vi "ReadEXCEL.vi"(8 "错误输入（无错误）":errorcluster, 9 "EXCEL 标签":string="Sheet1", 10 "路径":path) -> (0 "错误输出":errorcluster, 1 "数据":string[][](array[string]))   [LabVIEW 2018]
panel:
  in  "数组":string[][](array[string])
  in  "Excel._Worksheet":refnum<k7>
  in  "Excel._Application":refnum<k7>
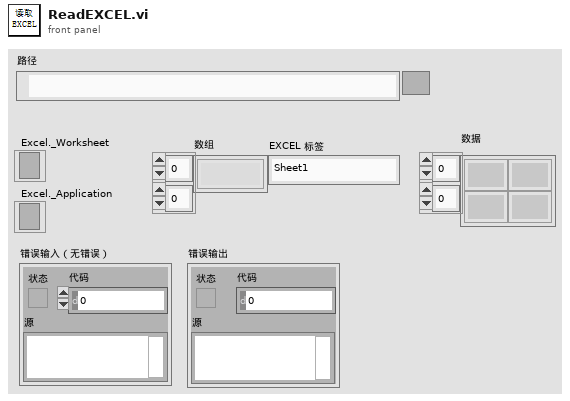
[diagram p1: front panel]
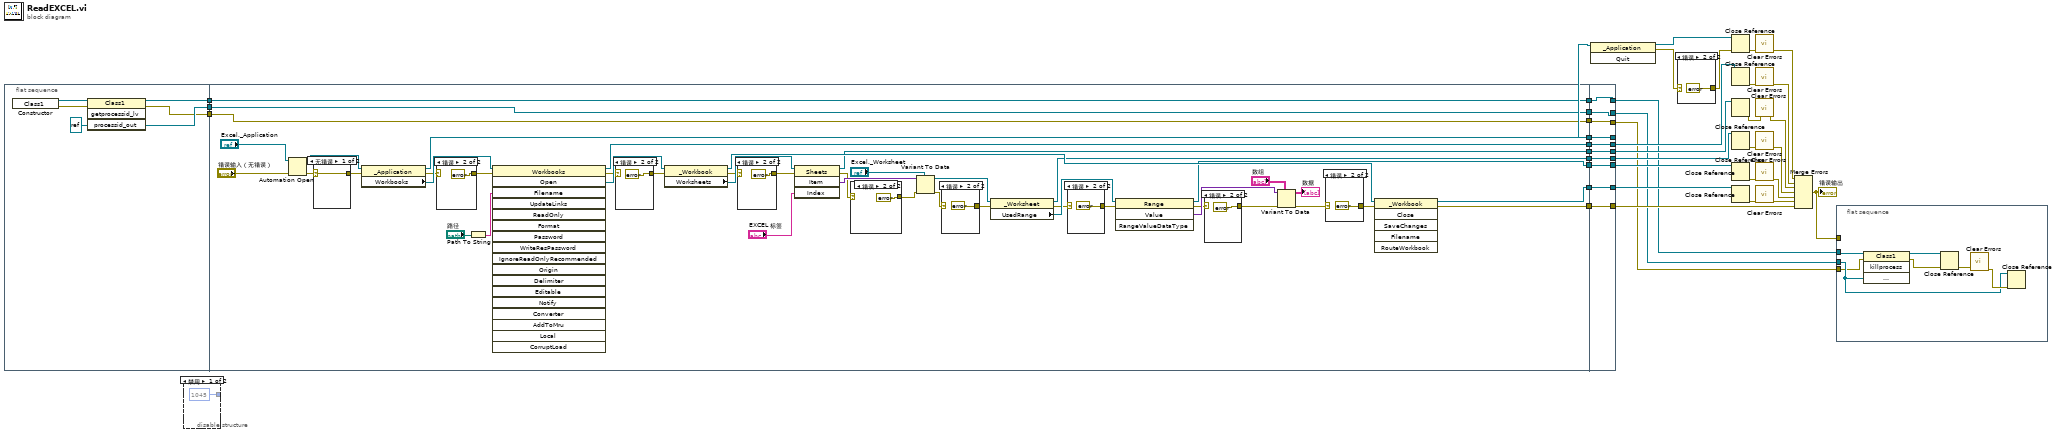
[diagram p0: block diagram]
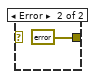
[diagram p11: hidden frame]
diagram:
  n1 = flat-sequence {
    tunnel: [w43] -> w11
    tunnel: [w42] -> w10
    tunnel: [w40] -> w3
    tunnel: [w75] -> w18
    tunnel: [w74] -> w17
    tunnel: [w73] -> w16
    tunnel: [w68] -> w15
    tunnel: [w70] -> w14
    tunnel: [w72] -> w13
    tunnel: [w71] -> w12
    tunnel: w11 -> [w47]
    tunnel: w10 -> [w48]
    tunnel: [w48] -> w9
    tunnel: [w47] -> w8
    tunnel: [w46] -> w4
    tunnel: w3 -> [w46]
    tunnel: [w112] -> w22
    tunnel: [w113] -> w29
    tunnel: [w114] -> w1
    tunnel: [w115] -> w31
    tunnel: [w116] -> w33
    tunnel: [w117] -> w35
    tunnel: [w118] -> w36
    tunnel: w18 -> [w118]
    tunnel: w17 -> [w117]
    tunnel: w16 -> [w116]
    tunnel: w15 -> [w115]
    tunnel: w14 -> [w114]
    tunnel: w13 -> [w113]
    tunnel: w12 -> [w112]
    tunnel: [w111] -> w5
    tunnel: w9 -> [w111]
    tunnel: [w110] -> w6
    tunnel: w8 -> [w110]
    tunnel: [w109] -> w2
    tunnel: w4 -> [w109]
    frame #0 {
      n2 = constructor class="Class1"() -> (reference out=w45:refnum<k24>, error out=w41:errorcluster)  [unwired: 3 in, 1 out]
      n3 = invoke on="调用节点" class="Class1" method="getprocessid_lv"(reference=w45, error in=w41, "processid_out"=refnum<k24> refnum) -> (reference out=w43:refnum<k24>, error out=w40:errorcluster, "processid_out"=w42:refnum<k24>)  [unwired: 1 in, 1 out]
    }
    frame #1 {
      n4 = Automation Open(error in (no error)="错误输入（无错误）", Automation Refnum="Excel._Application") -> (Automation Refnum=w69:refnum<k7>, error out=w66:errorcluster)  [unwired: 2 out]
      n5 = case shown="无错误" w66 {
        selector: w66 -> [w107 _]
        tunnel: [w107 errorcluster {"status"=FALSE, "code"=0, "source"=""} ("error IO")] -> w65
        frame No Error {
        }
        frame Error {
        }
      }
      n6 = property class="_Application"(reference=w69, error in=w65) -> (reference out=w70:refnum<k7>, error out=w64:errorcluster, "Workbooks"=w67:refnum<k7>)
      n7 = case shown="错误" w64 {
        selector: w64 -> [w105 _]
        tunnel: [w105 errorcluster {"status"=FALSE, "code"=0, "source"=""} ("error IO")] -> w63
        frame No Error {
        }
        frame Error {
        }
      }
      n8 = Path To String(path="路径") -> (string=w79:string)
      n9 = invoke class="Workbooks" method="Open"(reference=w67, error in=w63, "Filename"=w79) -> (reference out=w68:refnum<k7>, error out=w62:errorcluster, "Open"=w90:refnum<k7>)  [unwired: 15 in, 15 out]
      n10 = case shown="错误" w62 {
        selector: w62 -> [w103 _]
        tunnel: [w103 errorcluster {"status"=FALSE, "code"=0, "source"=""} ("error IO")] -> w61
        frame No Error {
        }
        frame Error {
        }
      }
      n11 = property class="_Workbook"(reference=w90, error in=w61) -> (reference out=w78:refnum<k7>, error out=w60:errorcluster, "Worksheets"=w89:refnum<k7>)
      n12 = case shown="错误" w60 {
        selector: w60 -> [w101 _]
        tunnel: [w101 errorcluster {"status"=FALSE, "code"=0, "source"=""} ("error IO")] -> w59
        frame No Error {
        }
        frame Error {
        }
      }
      n13 = invoke class="Sheets" method="Item"(reference=w89, error in=w59, "Index"="EXCEL 标签") -> (reference out=w73:refnum<k7>, error out=w58:errorcluster, "Item"=w88:variant)  [unwired: 1 in, 1 out]
      n14 = case shown="错误" w58 {
        selector: w58 -> [w99 _]
        tunnel: [w99 errorcluster {"status"=FALSE, "code"=0, "source"=""} ("error IO")] -> w57
        frame No Error {
        }
        frame Error {
        }
      }
      n15 = Variant To Data(error in=w57, type="Excel._Worksheet", Variant=w88) -> (data=w86:refnum<k7>, error out=w56:errorcluster)
      n16 = case shown="错误" w56 {
        selector: w56 -> [w97 _]
        tunnel: [w97 errorcluster {"status"=FALSE, "code"=0, "source"=""} ("error IO")] -> w55
        frame No Error {
        }
        frame Error {
        }
      }
      n17 = property class="_Worksheet"(reference=w86, error in=w55) -> (reference out=w74:refnum<k7>, error out=w54:errorcluster, "UsedRange"=w85:refnum<k7>)
      n18 = case shown="错误" w54 {
        selector: w54 -> [w95 _]
        tunnel: [w95 errorcluster {"status"=FALSE, "code"=0, "source"=""} ("error IO")] -> w53
        frame No Error {
        }
        frame Error {
        }
      }
      n19 = invoke class="Range" method="Value"(reference=w85, error in=w53) -> (reference out=w75:refnum<k7>, error out=w52:errorcluster, "Value"=w84:variant)  [unwired: 2 in, 1 out]
      n20 = case shown="错误" w52 {
        selector: w52 -> [w93 _]
        tunnel: [w93 errorcluster {"status"=FALSE, "code"=0, "source"=""} ("error IO")] -> w51
        frame No Error {
        }
        frame Error {
        }
      }
      n21 = Variant To Data(error in=w51, type="数组", Variant=w84) -> (data=→"数据":string[][], error out=w50:errorcluster)
      n22 = case shown="错误" w50 {
        selector: w50 -> [w91 _]
        tunnel: [w91 errorcluster {"status"=FALSE, "code"=0, "source"=""} ("error IO")] -> w49
        frame No Error {
        }
        frame Error {
        }
      }
      n23 = invoke class="_Workbook" method="Close"(reference=w78, error in=w49) -> (reference out=w72:refnum<k7>, error out=w71:errorcluster)  [unwired: 4 in, 4 out]
    }
    frame #2 {
    }
  }
  n24 = disable-structure shown="禁用" {
    disable-tunnel: [1045 ("specific error code to clear (0: all)") _] -> _
    frame Disabled {
    }
    frame Enabled {
    }
  }
  n25 = invoke class="_Application" method="Quit"(reference=w1) -> (reference out=w21:refnum<k7>, error out=w20:errorcluster)  [unwired: 2 in, 1 out]
  n26 = case shown="错误" w20 {
    selector: w20 -> [w120 _]
    tunnel: [w120 errorcluster {"status"=FALSE, "code"=0, "source"=""} ("error IO")] -> w19
    frame No Error {
    }
    frame Error {
    }
  }
  n27 = Close Reference(reference=w21, error in (no error)=w19) -> (error out=w30:errorcluster)
  n28 = Close Reference(reference=w31) -> (error out=w32:errorcluster)  [unwired: 1 in]
  n29 = Close Reference(reference=w33) -> (error out=w34:errorcluster)  [unwired: 1 in]
  n30 = Close Reference(reference=w35) -> (error out=w37:errorcluster)  [unwired: 1 in]
  n31 = Close Reference(reference=w36) -> (error out=w38:errorcluster)  [unwired: 1 in]
  n32 = Close Reference(reference=w29) -> (error out=w39:errorcluster)  [unwired: 1 in]
  n33 = call <vilib>:"Clear Errors.vi"("error in (no error)"=w30) -> ("error out"=w28:errorcluster)  [unwired: 5 in, 1 out]
  n34 = call <vilib>:"Clear Errors.vi"("error in (no error)"=w32) -> ("error out"=w27:errorcluster)  [unwired: 5 in, 1 out]
  n35 = call <vilib>:"Clear Errors.vi"("error in (no error)"=w34) -> ("error out"=w26:errorcluster)  [unwired: 5 in, 1 out]
  n36 = call <vilib>:"Clear Errors.vi"("error in (no error)"=w37) -> ("error out"=w25:errorcluster)  [unwired: 5 in, 1 out]
  n37 = call <vilib>:"Clear Errors.vi"("error in (no error)"=w38) -> ("error out"=w24:errorcluster)  [unwired: 5 in, 1 out]
  n38 = call <vilib>:"Clear Errors.vi"("error in (no error)"=w39) -> ("error out"=w23:errorcluster)  [unwired: 5 in, 1 out]
  n39 = Merge Errors(w28, w27, w26, w25, w24, w23, w22) -> (w7:errorcluster)
  "错误输出" <- w7
  n40 = flat-sequence {
    tunnel: w7 -> [_]
    tunnel: w6 -> [w128]
    tunnel: w5 -> [w123]
    tunnel: w2 -> [w122]
    frame #0 {
      n41 = invoke on="调用节点" class="Class1" method="killprocess"(reference=w128, error in=w122, "processid"=w123) -> (reference out=w127:refnum<k24>, error out=w126:errorcluster)  [unwired: 1 in, 2 out]
      n42 = Close Reference(reference=w127, error in (no error)=w126) -> (error out=w125:errorcluster)
      n43 = call <vilib>:"Clear Errors.vi"("error in (no error)"=w125) -> ("error out"=w124:errorcluster)  [unwired: 5 in, 1 out]
      n44 = Close Reference(reference=w123, error in (no error)=w124) -> ()  [unwired: 1 out]
    }
  }
